vi "LAN Apply Settings.vi"(8 "error in":errorcluster, 10 "Node In":string, 11 "VISA resource name":refnum<visa-resource-name>) -> (0 "error out":errorcluster, 2 "Node Out":string, 3 "VISA resource name out":refnum<visa-resource-name>, 4 "Command String":string)   [LabVIEW 2012, in "Keithley 2600 Series.lvlib"]
doc: "This VI applies the configured LAN settings.\n\n<b>Note:</b> If you are connected to the instrument by LAN, this will cause you to lose connection.\n\n<b>Functions and Attributes Used</b>\nlan.applysettings()"
uses:
  Keithley 2600 Series.lvlib
panel:
  # "(c) 2008 Keithley Instruments, Inc.  ALL RIGHTS RESERVED."
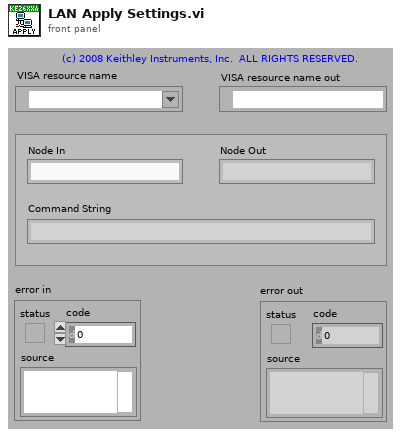
[diagram p1: front panel]
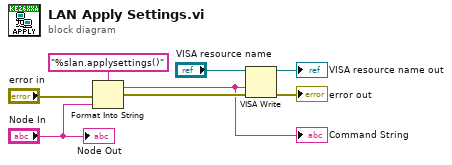
[diagram p0: block diagram]
diagram:
  n1 = Format Into String(format string="%slan.applysettings()", error in="error in", "Node In") -> (resulting string=w3:string, error out=w6:errorcluster)  [unwired: 1 in]
  "Command String" <- w3
  n2 = VISA Write(VISA resource name="VISA resource name", write buffer=w3, error in (no error)=w6) -> (VISA resource name out=→"VISA resource name out":refnum<visa-resource-name>, error out=→"error out":errorcluster)  [unwired: 1 out]
  "Node Out" <- "Node In"
